vi "Dynamic Main.vi"(8 "错误输入（无错误）":errorcluster, 11 "UserInfo":string="UserInfo") -> (0 "错误输出":errorcluster)   [LabVIEW 2011]
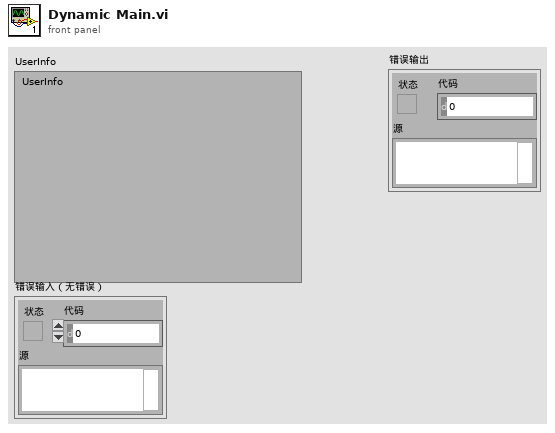
[diagram p1: front panel]
types:
  T1 = enum32{"Invalid", "Standard", "Closed", "Hidden", "Minimized", "Maximized"}
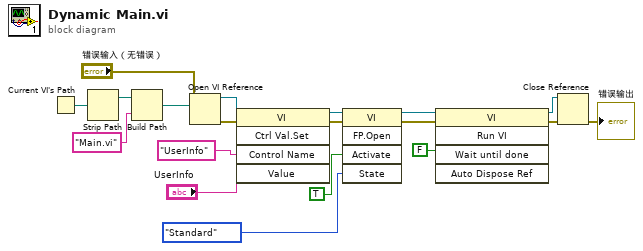
[diagram p0: block diagram]
diagram:
  n1 = Current VI's Path() -> (path=w18:path)
  n2 = Strip Path(path=w18) -> (stripped path=w13:path)  [unwired: 1 out]
  n3 = Build Path(base path=w13, name or relative path="Main.vi" ("名称或相对路径")) -> (appended path=w19:path)
  n4 = Open VI Reference(vi path=w19, error in (no error)="错误输入（无错误）") -> (vi reference=w16:refnum<vi>, error out=w14:errorcluster)  [unwired: 4 in]
  n5 = invoke class="VI" method="Ctrl Val.Set"(reference=w16, error in=w14, "Control Name"="UserInfo" ("控件名"), "Value"="UserInfo") -> (reference out=w7:refnum<vi>, error out=w6:errorcluster)  [unwired: 1 in, 3 out]
  n6 = invoke class="VI" method="FP.Open"(reference=w7, error in=w6, "Activate"=TRUE ("激活？"), "State"=T1."Standard" ("州")) -> (reference out=w11:refnum<vi>, error out=w10:errorcluster)  [unwired: 1 in, 3 out]
  n7 = invoke class="VI" method="Run VI"(reference=w11, error in=w10, "Wait until done"=FALSE ("结束前等待")) -> (reference out=w9:refnum<vi>, error out=w8:errorcluster)  [unwired: 2 in, 3 out]
  n8 = Close Reference(reference=w9, error in (no error)=w8) -> (error out=→"错误输出":errorcluster)
